vi "Flat Sequence Structure Test.vi"   [LabVIEW 2019]
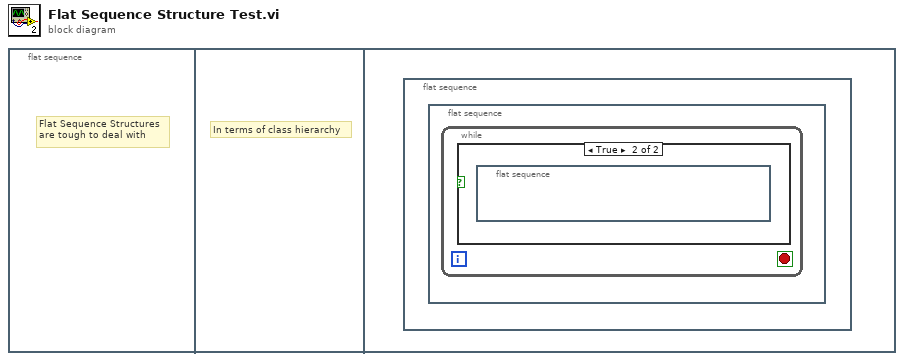
[diagram p0: block diagram]
diagram:
  n1 = flat-sequence {
    frame #0 {
      # "Flat Sequence Structures\nare tough to deal with"
    }
    frame #1 {
      # "In terms of class hierarchy"
    }
    frame #2 {
      n2 = flat-sequence {
        frame #0 {
          n3 = flat-sequence {
            frame #0 {
              n4 = while {
                stop <- _ stop-if-true
                n5 = case shown="True" {
                  selector: _ -> [_ _]
                  frame False {
                  }
                  frame True {
                    n6 = flat-sequence {
                      frame #0 {
                      }
                    }
                  }
                }
              }
            }
          }
        }
      }
    }
  }
